vi "Verify.vi"(5 "Options":T1, 6 "Extension(txt)":string="txt", 7 "Test VI (caller)":string, 8 "error in":errorcluster, 10 "Anything":variant) -> (0 "error out":errorcluster, 1 "Failure Message":string, 2 "Passed?":bool)   [LabVIEW 2020, in "Approval Tests.lvlib"]
doc: "Performs an approval test.\n\nThe first call, the test passes and the test data is written to the approved file.\n\nOn subsequent runs the test data is compared to the contents of the approved file.\nIf it is a match, the test passes.\nIf it is not a match, the test fails and the test data is written to the actual file.\n\nAt the point the user can diff the approved and actual files and determine if they approve of the changes or not. If they approve, they replace the old approved file with the actual file. \n\nNOTE: You should keep the approved files in Source Code Control. You should ignore *.actual in your .gitignore file - there is no need to store those."
uses:
  Approval Tests.lvlib
  Options.ctl
  Reporter/Reporter.lvclass
  Printer/Printer.lvclass
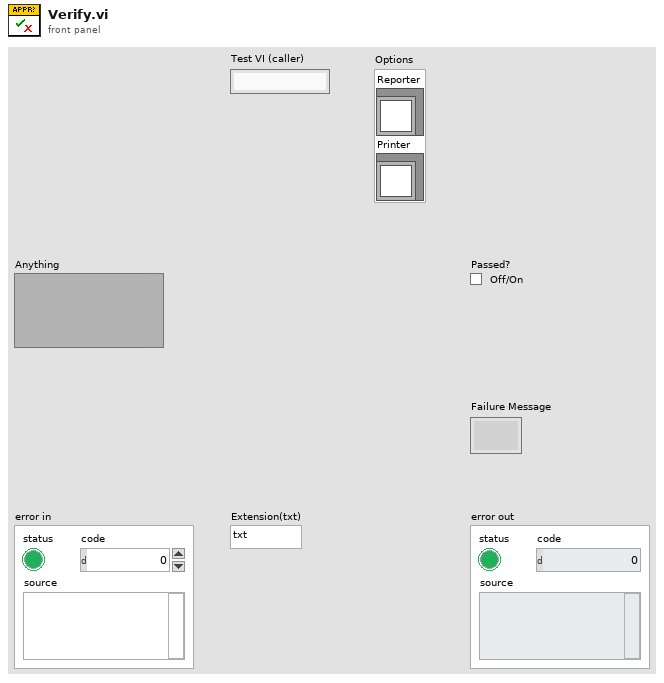
[diagram p1: front panel]
types:
  T1 = typedef "Approval Tests.lvlib/Options.ctl" = cluster{"Reporter":refnum<class "Reporter.lvclass">, "Printer":refnum<class "Printer.lvclass">}
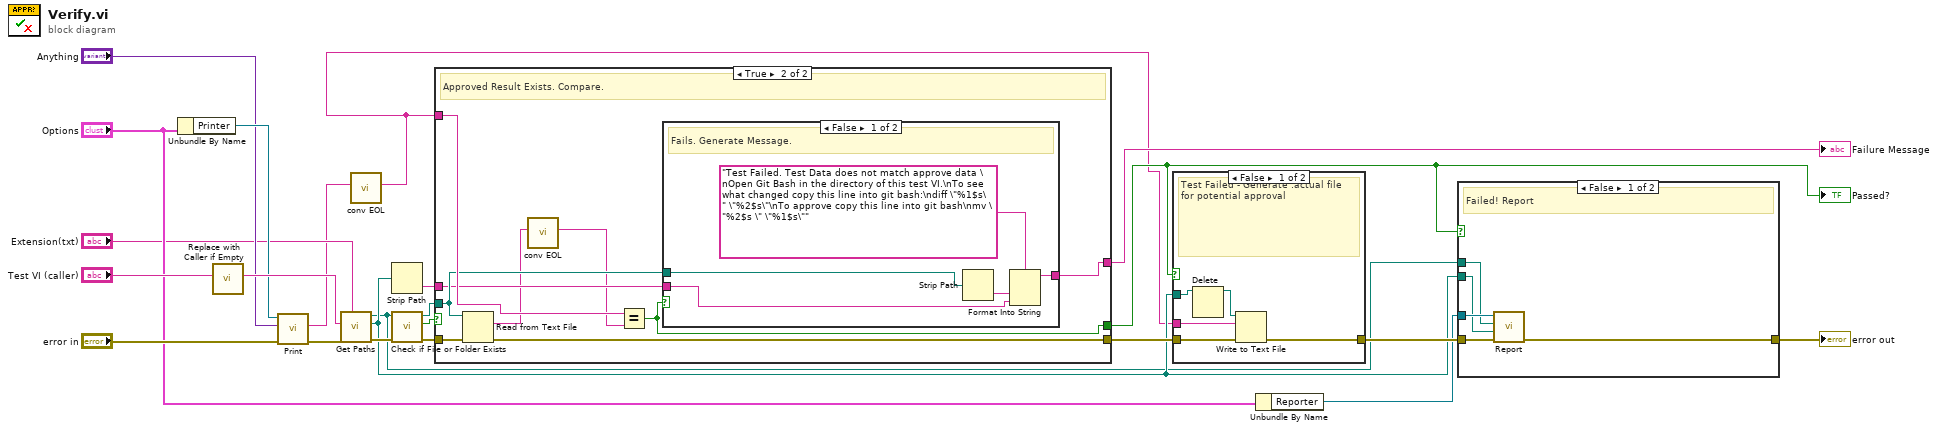
[diagram p0: block diagram]
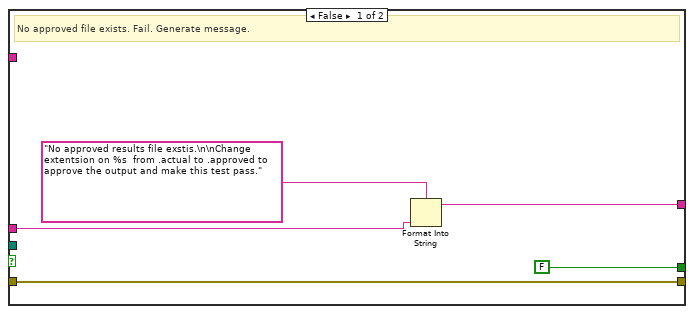
[diagram p4: hidden frame]
diagram:
  n1 = Unbundle By Name("Options") -> ("Printer"=w5:refnum<class "Printer.lvclass">)
  n2 = call "Replace with Caller if Empty.vi"("Test VI (caller) in"="Test VI (caller)") -> ("Test VI (caller) out"=w8:string)  [unwired: 10 in]
  n3 = call-dynamic "Print.vi"("error in"="error in", "Anything In"="Anything", "Printer in"=w5) -> ("error out"=w17:errorcluster, "Printed String"=w2:string)  [unwired: 6 in, 1 out]
  n4 = call "Get Paths.vi"("Extension(txt)"="Extension(txt)", "error in"=w17, "VI name"=w8) -> ("error out"=w23:errorcluster, "recived path"=w11:path, "approved path"=w10:path)  [unwired: 6 in]
  n5 = call "conv EOL.vi"("standard output in"=w2) -> ("result string"=w1:string)  [unwired: 10 in]
  n6 = Strip Path(path=w11) -> (name=w13:string)  [unwired: 1 out]
  n7 = call <vilib>:"Check if File or Folder Exists.vi"("error in (no error)"=w23, "path"=w10) -> ("error out"=w22:errorcluster, "file or folder exists?"=w15:bool, "dup path"=w16:path)  [unwired: 7 in]
  n8 = case shown="True" w15 {
    tunnel: w1 -> [_ w34]
    tunnel: [w28 w36] -> w21
    tunnel: w22 -> [w28 w37]
    tunnel: w16 -> [_ w32]
    tunnel: [FALSE ("Passed?") w35] -> w12
    tunnel: [w24 w33] -> w14
    tunnel: w13 -> [w26 w31]
    frame False {
      # "No approved file exists. Fail. Generate message."
      n9 = Format Into String(format string="No approved results file exstis.\n\nChange extentsion on %s  from .actual to .approved to approve the output and make this test pass.", w26) -> (resulting string=w24:string)  [unwired: 2 in, 1 out]
    }
    frame True {
      # "Approved Result Exists. Compare."
      n10 = Read from Text File(file (use dialog)=w32, error in=w37) -> (text=w30:string, error out=w36:errorcluster)  [unwired: 2 in, 2 out]
      n11 = call "conv EOL.vi"("standard output in"=w30) -> ("result string"=w29:string)  [unwired: 10 in]
      n12 = Equal?(x=w34, y=w29) -> (x = y?=w35:bool)
      n13 = case shown="False" w35 {
        tunnel: [w42 _] -> w33
        tunnel: w32 -> [w39 _]
        tunnel: w31 -> [w38 _]
        frame False {
          # "Fails. Generate Message."
          n14 = Strip Path(path=w39) -> (name=w40:string)  [unwired: 1 out]
          n15 = Format Into String(format string="Test Failed. Test Data does not match approve data \nOpen Git Bash in the directory of this test VI.\nTo see what changed copy this line into git bash:\ndiff \"%1$s\" \"%2$s\"\nTo approve copy this line into git bash\nmv \"%2$s \" \"%1$s\"", w40, w38) -> (resulting string=w42:string)  [unwired: 2 in, 1 out]
        }
        frame True {
          # "Passes. No Message Needed.."
        }
      }
    }
  }
  "Passed?" <- w12
  "Failure Message" <- w14
  n16 = case shown="False" w12 {
    tunnel: w21 -> [w46 w48]
    tunnel: [w47 w48] -> w20
    tunnel: w11 -> [w45 _]
    tunnel: w1 -> [w43 _]
    frame False {
      # "Test Failed - Generate .actual file for potential approval"
      n17 = Delete(path (use dialog)=w45) -> (deleted path=w44:path)  [unwired: 4 in, 2 out]
      n18 = Write to Text File(file (use dialog)=w44, text=w43, error in=w46) -> (error out=w47:errorcluster)  [unwired: 1 in, 2 out]
    }
    frame True {
      # "Passed - no need for .actual file"
    }
  }
  n19 = Unbundle By Name("Options") -> ("Reporter"=w7:refnum<class "Reporter.lvclass">)
  n20 = case shown="False" w12 {
    tunnel: w11 -> [w49 _]
    tunnel: w10 -> [w50 _]
    tunnel: w7 -> [w51 _]
    tunnel: w20 -> [w53 w54]
    tunnel: [w52 w54] -> w19
    frame False {
      # "Failed! Report"
      n21 = call-dynamic "Report.vi"("error in"=w53, "Received"=w49, "Approved"=w50, "Reporter in"=w51) -> ("error out"=w52:errorcluster)  [unwired: 5 in, 2 out]
    }
    frame True {
      # "Passed - Nothing to Report"
    }
  }
  "error out" <- w19
